vi "DatabaseManager.vi"() -> ()   [LabVIEW 2018]
uses:
  <vilib>/addons/database/Connection.llb/DB Tools Open Connec (String).vi
  <vilib>/addons/database/Connection.llb/Conn Execute.vi
  <vilib>/addons/database/Recordset.llb/Rec Fetch Recordset Data (R).vi
  <vilib>/addons/database/Recordset.llb/Rec Destroy - Connection.vi
  <vilib>/addons/database/NI_Database_API.lvlib
panel:
  in  "测试数据库（服务器）":bool
  in  "密码":string
  in  "用户名称":string
  in  "服务器名称（服务器）":string
  in  "在服务器上选择数据库（服务器）":u16(ring)
  in  "取消":bool
  in  "确定":bool
  # "请输入登陆服务器信息："
  # "在服务器上选择数据库"
  # "密码"
  # "用户名称"
  # "请输入服务器名称："
  # "服务器名称"
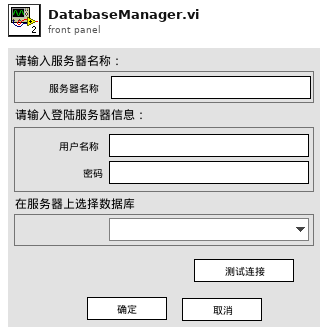
[diagram p1: front panel]
types:
  T1 = enum16{"open", "replace", "create", "open or create", "replace or create", "replace or create with confirmation"}
  T2 = typedef "NI_Database_API.lvlib/Conn ObjectReference.ctl" = refnum<k1>
  T3 = typedef "NI_Database_API.lvlib/Rec ObjectReference.ctl" = refnum<k1>
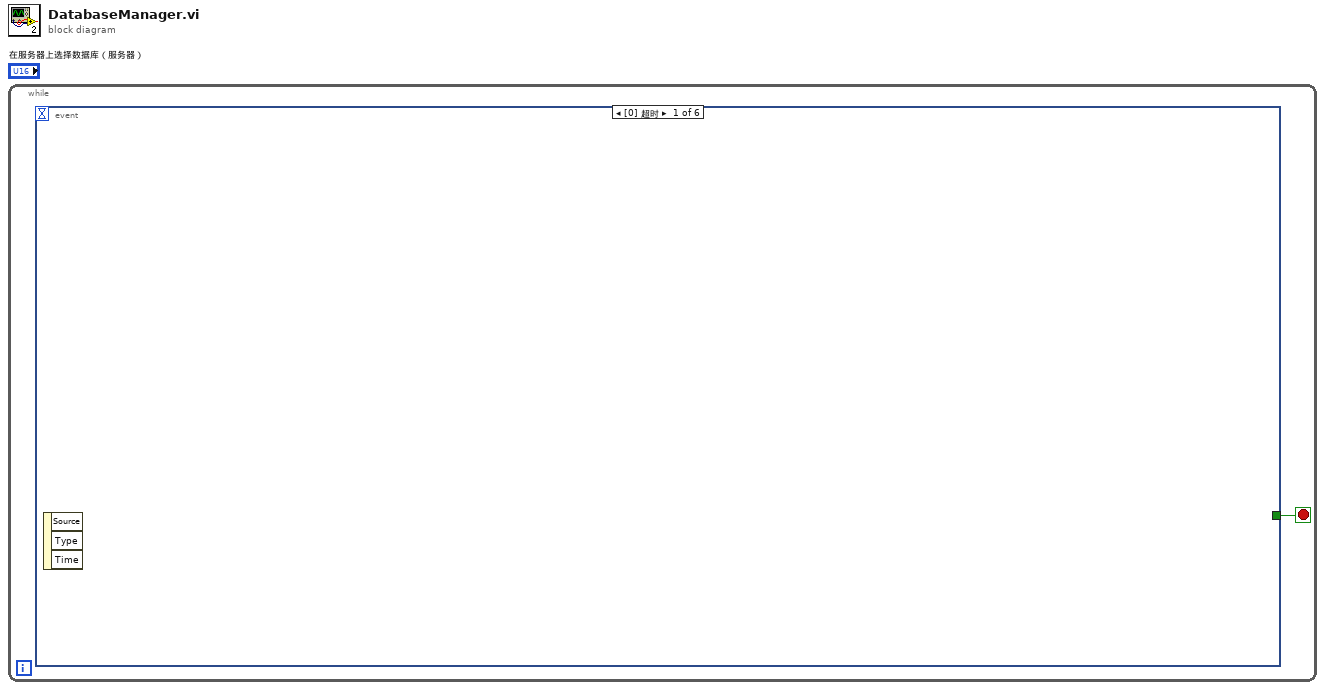
[diagram p0: block diagram]
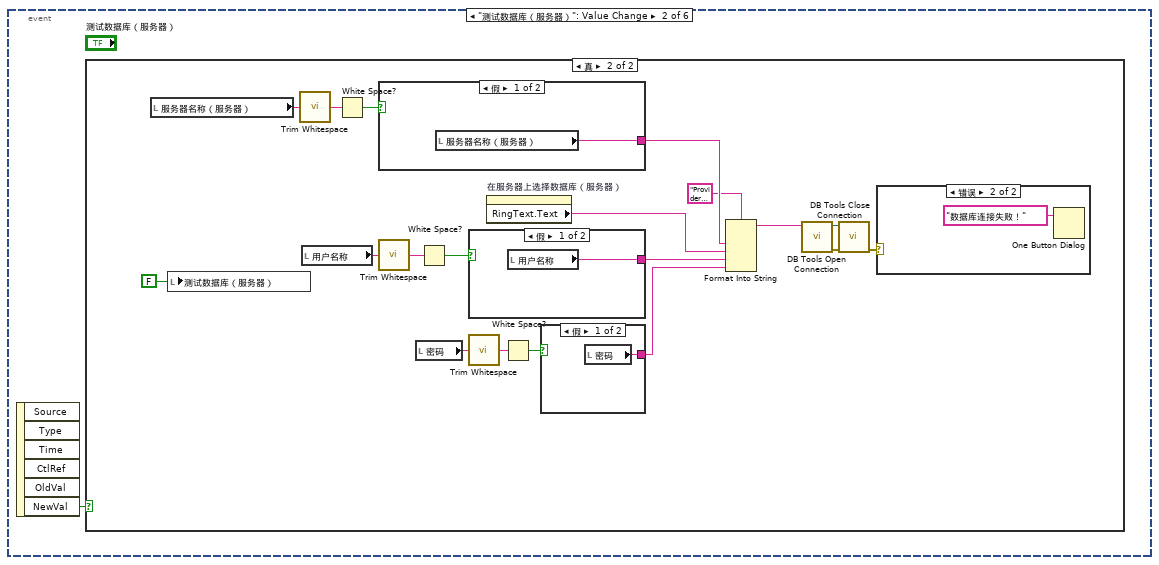
[diagram p2: hidden frame]
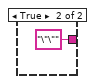
[diagram p4: hidden frame]
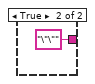
[diagram p5: hidden frame]
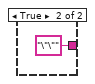
[diagram p6: hidden frame]
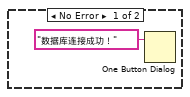
[diagram p7: hidden frame]
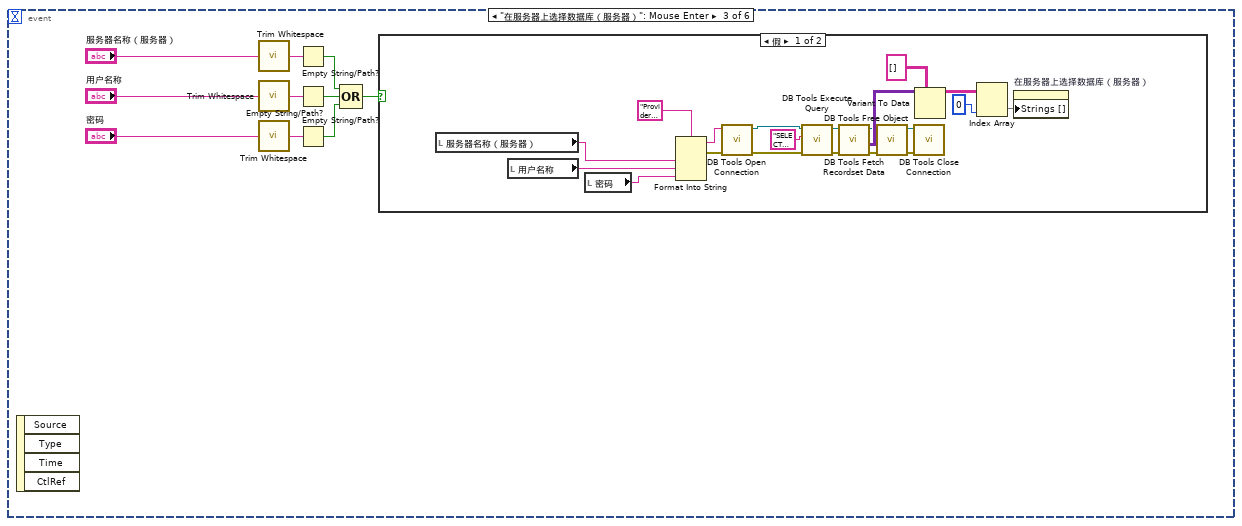
[diagram p8: hidden frame]
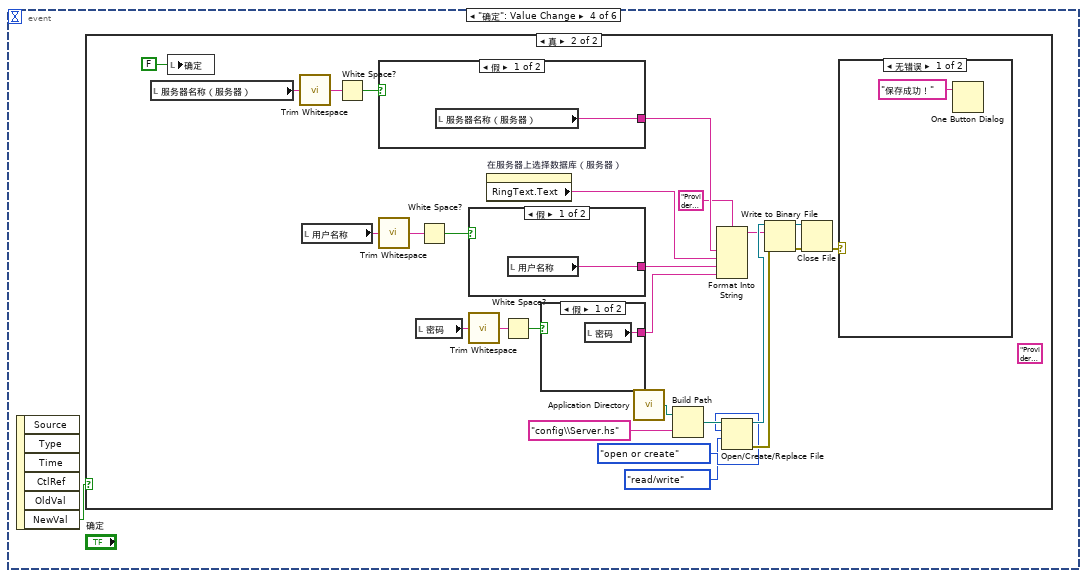
[diagram p10: hidden frame]
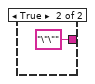
[diagram p13: hidden frame]
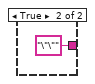
[diagram p14: hidden frame]
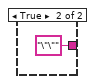
[diagram p15: hidden frame]
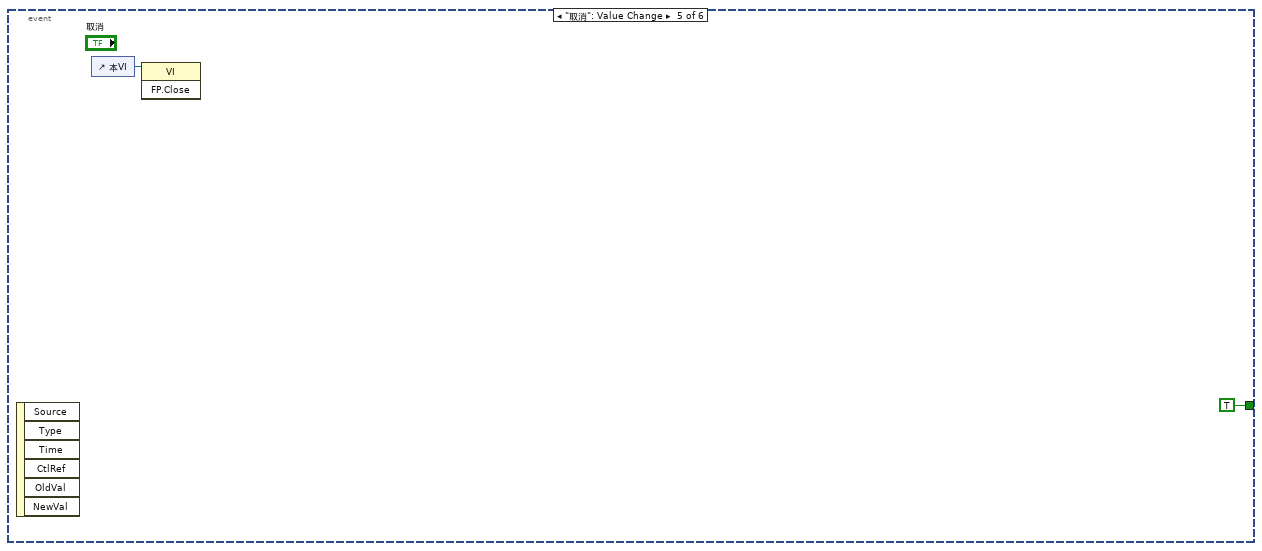
[diagram p16: hidden frame]
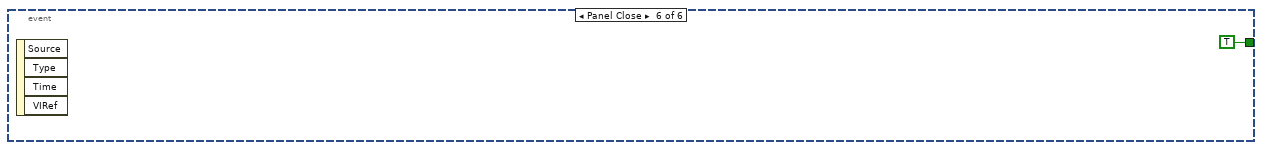
[diagram p17: hidden frame]
diagram:
  n1 = while {
    stop <- w1 stop-if-true
    n2 = event shown="[0] 超时" {
      selector: _ -> [_ _ _ _ _ _]
      dyn-events: _ -> [_ _ _ _ _ _]
      timeout: _ -> [_ _ _ _ _ _]
      tunnel: [_ _ _ _ TRUE TRUE] -> w1
      event Timeout {
        n3 = event-data() -> ()  [unwired: 1 in, 3 out]
      }
      event "测试数据库（服务器）": Value Change {
        n4 = event-data() -> ("NewVal"=w2:bool)  [unwired: 1 in, 5 out]
        n5 = case shown="真" w2 {
          frame False {
          }
          frame True {
            n6 = local read "服务器名称（服务器）"() -> (w17:string)
            n7 = local write "测试数据库（服务器）"(FALSE ("测试数据库（服务器）")) -> ()
            n8 = call <vilib>:"Trim Whitespace.vi"("string"=w17) -> ("trimmed string"=w15:string)  [unwired: 1 in]
            n9 = local read "用户名称"() -> (w12:string)
            n10 = White Space?(1:w15) -> (0:w16:bool)
            n11 = case shown="假" w16 {
              tunnel: [w26 "\"\""] -> w14
              frame False {
                n12 = local read "服务器名称（服务器）"() -> (w26:string)
              }
              frame True {
              }
            }
            n13 = call <vilib>:"Trim Whitespace.vi"("string"=w12) -> ("trimmed string"=w8:string)  [unwired: 1 in]
            n14 = local read "密码"() -> (w13:string)
            n15 = White Space?(1:w8) -> (0:w9:bool)
            n16 = case shown="假" w9 {
              tunnel: [w24 "\"\""] -> w7
              frame False {
                n17 = local read "用户名称"() -> (w24:string)
              }
              frame True {
              }
            }
            n18 = call <vilib>:"Trim Whitespace.vi"("string"=w13) -> ("trimmed string"=w10:string)  [unwired: 1 in]
            n19 = property on="在服务器上选择数据库（服务器）" class="Ring (严格)"() -> ("RingText.Text"=w3:string)  [unwired: 2 in, 2 out]
            n20 = White Space?(1:w10) -> (0:w11:bool)
            n21 = case shown="假" w11 {
              tunnel: [w22 "\"\""] -> w6
              frame False {
                n22 = local read "密码"() -> (w22:string)
              }
              frame True {
              }
            }
            n23 = Format Into String(format string="Provider=SQLOLEDB.1;Persist Security Info=True;Data Source=%s;Initial Catalog=%s;User ID=%s;Password=%s" ("格式字符串"), w14, w3, w7, w6) -> (resulting string=w4:string)  [unwired: 2 in, 1 out]
            n24 = call-poly <vilib>:"DB Tools Open Connection.vi"("connection information"=w4) -> ("error out"=w19:errorcluster, "connection reference"=w20:T2)  [unwired: 7 in]
            n25 = call <vilib>:"DB Tools Close Connection.vi"("error in (no error)"=w19, "connection reference"=w20) -> ("error out"=w18:errorcluster)  [unwired: 5 in]
            n26 = case shown="错误" w18 {
              frame No Error {
                n27 = One Button Dialog(message="数据库连接成功！" ("消息")) -> ()  [unwired: 1 in, 1 out]
              }
              frame Error {
                n28 = One Button Dialog(message="数据库连接失败！" ("消息")) -> ()  [unwired: 1 in, 1 out]
              }
            }
          }
        }
      }
      event "在服务器上选择数据库（服务器）": Mouse Enter {
        n29 = event-data() -> ()  [unwired: 1 in, 4 out]
        n30 = call <vilib>:"Trim Whitespace.vi"("string"="服务器名称（服务器）") -> ("trimmed string"=w36:string)  [unwired: 1 in]
        n31 = call <vilib>:"Trim Whitespace.vi"("string"="用户名称") -> ("trimmed string"=w35:string)  [unwired: 1 in]
        n32 = call <vilib>:"Trim Whitespace.vi"("string"="密码") -> ("trimmed string"=w34:string)  [unwired: 1 in]
        n33 = Empty String/Path?(string/path=w36) -> (empty?=w33:bool)
        n34 = Empty String/Path?(string/path=w35) -> (empty?=w32:bool)
        n35 = Empty String/Path?(string/path=w34) -> (empty?=w31:bool)
        n36 = Compound Arithmetic op=OR ("复合运算")(w33, w32, w31) -> (w30:bool)
        n37 = case shown="假" w30 {
          frame False {
            n38 = local read "服务器名称（服务器）"() -> (w43:string)
            n39 = local read "用户名称"() -> (w42:string)
            n40 = local read "密码"() -> (w41:string)
            n41 = Format Into String(format string="Provider=SQLOLEDB.1;Persist Security Info=False;Data Source=%s;User ID=%s;Password=%s" ("格式字符串"), w43, w42, w41) -> (resulting string=w58:string, error out=w44:errorcluster)  [unwired: 2 in]
            n42 = call-poly <vilib>:"DB Tools Open Connection.vi"("error in (no error)"=w44, "connection information"=w58) -> ("error out"=w49:errorcluster, "connection reference"=w57:T2)  [unwired: 6 in]
            n43 = call-poly <vilib>:"DB Tools Execute Query.vi"("error in (no error)"=w49, "SQL query"="SELECT Name FROM Master..SysDatabases where dbid>6 ORDER BY Name", "connection reference"=w57) -> ("error out"=w56:errorcluster, "recordset reference"=w55:T3)  [unwired: 5 in]
            n44 = call-poly <vilib>:"DB Tools Fetch Recordset Data.vi"("error in (no error)"=w56, "recordset reference"=w55) -> ("error out"=w47:errorcluster, "recordset data"=w54:variant[][], "recordset reference out"=w48:T3)  [unwired: 3 in]
            n45 = call-poly <vilib>:"DB Tools Free Object.vi"("error in (no error)"=w47, "recordset reference"=w48) -> ("error out"=w46:errorcluster, "connection reference"=w45:T2)  [unwired: 8 in]
            n46 = call <vilib>:"DB Tools Close Connection.vi"("error in (no error)"=w46, "connection reference"=w45) -> ()  [unwired: 5 in, 1 out]
            n47 = Variant To Data(type=string[][] [] ("字符串[]"), Variant=w54) -> (data=w52:string[][])  [unwired: 1 in, 1 out]
            n48 = Index Array(array=w52, index (col)=0 ("禁用的索引 (列)")) -> (element=w51:string[])  [unwired: 1 in]
            n49 = property on="在服务器上选择数据库（服务器）" class="Ring (严格)"("Strings []"=w51) -> ()  [unwired: 2 in, 2 out]
          }
          frame True {
          }
        }
      }
      event "确定": Value Change {
        n50 = event-data() -> ("NewVal"=w60:bool)  [unwired: 1 in, 5 out]
        n51 = case shown="真" w60 {
          frame False {
          }
          frame True {
            (unwired) "Provider=SQLNCLI11.1;Integrated Security=SSPI;Persist Security Info=False;User ID=\"\";Initial Catalog=SanliServer;Data Source=(localdb)\\mssqllocaldb;Initial File Name=\"\";Server SPN=\"\""
            n52 = local read "服务器名称（服务器）"() -> (w86:string)
            n53 = local write "确定"(FALSE ("确定")) -> ()
            n54 = call <vilib>:"Trim Whitespace.vi"("string"=w86) -> ("trimmed string"=w84:string)  [unwired: 1 in]
            n55 = local read "用户名称"() -> (w81:string)
            n56 = White Space?(1:w84) -> (0:w85:bool)
            n57 = case shown="假" w85 {
              tunnel: [w92 "\"\""] -> w83
              frame False {
                n58 = local read "服务器名称（服务器）"() -> (w92:string)
              }
              frame True {
              }
            }
            n59 = call <vilib>:"Trim Whitespace.vi"("string"=w81) -> ("trimmed string"=w77:string)  [unwired: 1 in]
            n60 = local read "密码"() -> (w82:string)
            n61 = White Space?(1:w77) -> (0:w78:bool)
            n62 = case shown="假" w78 {
              tunnel: [w90 "\"\""] -> w76
              frame False {
                n63 = local read "用户名称"() -> (w90:string)
              }
              frame True {
              }
            }
            n64 = call <vilib>:"Trim Whitespace.vi"("string"=w82) -> ("trimmed string"=w79:string)  [unwired: 1 in]
            n65 = property on="在服务器上选择数据库（服务器）" class="Ring (严格)"() -> ("RingText.Text"=w69:string)  [unwired: 2 in, 2 out]
            n66 = White Space?(1:w79) -> (0:w80:bool)
            n67 = case shown="假" w80 {
              tunnel: [w88 "\"\""] -> w75
              frame False {
                n68 = local read "密码"() -> (w88:string)
              }
              frame True {
              }
            }
            n69 = call <vilib>:"Application Directory.vi"() -> ("Application Directory"=w73:path)
            n70 = Build Path(base path=w73, name or relative path="config\\Server.hs" ("名称或相对路径")) -> (appended path=w66:path)
            n71 = Format Into String(format string="Provider=SQLOLEDB.1;Persist Security Info=True;Data Source=%s;Initial Catalog=%s;User ID=%s;Password=%s" ("格式字符串"), w83, w69, w76, w75) -> (resulting string=w61:string)  [unwired: 2 in, 1 out]
            n72 = Open/Create/Replace File(file path (use dialog)=w66, operation (0:open)=T1."open or create" ("操作(0:open)"), access (0:read/write)=enum16{"read/write", "read-only", "write-only"}."read/write" ("权限(0:read/write)")) -> (refnum out=w68:refnum<file>, error out=w67:errorcluster)  [unwired: 3 in, 1 out]
            n73 = Write to Binary File(file (use dialog)=w68, data=w61, error in=w67) -> (refnum out=w71:refnum<file>, error out=w70:errorcluster)  [unwired: 3 in, 1 out]
            n74 = Close File(refnum=w71, error in=w70) -> (error out=w62:errorcluster)  [unwired: 1 out]
            n75 = case shown="无错误" w62 {
              frame No Error {
                n76 = One Button Dialog(message="保存成功！" ("消息")) -> ()  [unwired: 1 in, 1 out]
              }
              frame Error {
              }
            }
          }
        }
      }
      event "取消": Value Change {
        n77 = event-data() -> ()  [unwired: 1 in, 6 out]
        n78 = control-ref of="本VI"() -> (w94:refnum<vi>)
        n79 = invoke class="VI" method="FP.Close"(reference=w94) -> ()  [unwired: 2 in, 3 out]
      }
      event Panel Close {
        n80 = event-data() -> ()  [unwired: 1 in, 4 out]
      }
    }
  }
